vi "Key to Reference.vi"(8 "error in (no error)":errorcluster, 10 "Key":string, 11 "Edit.Subpanel in":refnum<class "Subpanel.Edit.lvclass">) -> (0 "error out":errorcluster, 2 "Reference":refnum<vi>, 3 "Edit.Subpanel out":refnum<class "Subpanel.Edit.lvclass">)   [LabVIEW 2019, in "Subpanel.Edit.lvclass"]
uses:
  Subpanel.Edit.lvclass
  Subpanel.Edit.lvclass/Subpanel.Edit.ctl
  Edit/Edit/Edit.lvclass
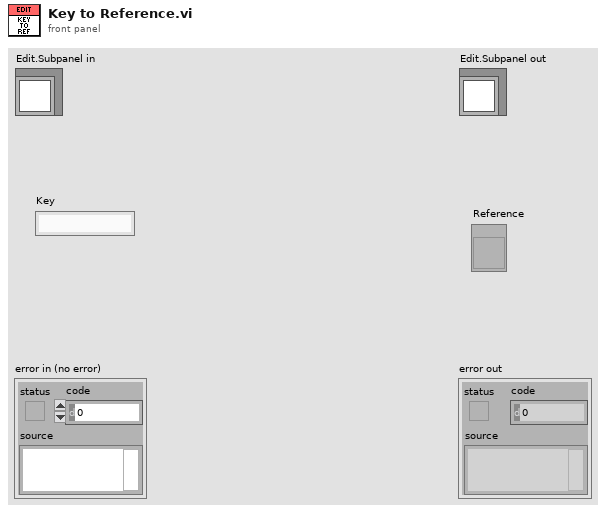
[diagram p1: front panel]
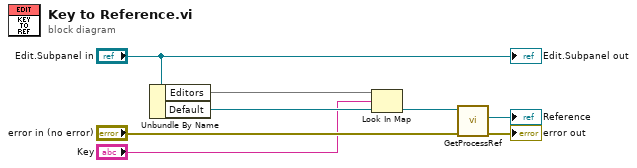
[diagram p0: block diagram]
diagram:
  n1 = Unbundle By Name("Edit.Subpanel in") -> ("Editors"=w2:map{string, refnum<class "Edit.lvclass">}, "Default"=w3:refnum<class "Edit.lvclass">)
  n2 = Look In Map(map=w2, key="Key", default value=w3) -> (value=w8:refnum<class "Edit.lvclass">)  [unwired: 1 out]
  n3 = call "GetProcessRef.vi"("error in (no error)"="error in (no error)", "Edit in"=w8) -> ("error out"=→"error out":errorcluster, "Static VI Ref"=→"Reference":refnum<vi>)  [unwired: 7 in, 1 out]
  "Edit.Subpanel out" <- "Edit.Subpanel in"
